vi "Actor Core.vi"(8 "error in":errorcluster, 11 "Image Averaging in":refnum<class "Image Averaging.lvclass">) -> (0 "error out":errorcluster, 3 "Actor out":refnum<class "Actor.lvclass">)   [LabVIEW 2022 SP3, in "Image Averaging.lvlib" / "Image Averaging.lvclass"]
doc: "(<B>Filename</B>: Actor Framework.lvlib:Actor.lvclass:Actor Core.vi)\n\nReceives messages to the actor, reacts to them, and initiates any error handling that may shut the actor down.\n\nDescendant classes may override this VI to append parallel tasks for the actor to complete while it handles messages. Overrides use the Call Parent Class Method node."
uses:
  Image Averaging.lvclass
  C:/Program Files/National Instruments/LabVIEW 2022/vi.lib/ActorFramework/Actor/Actor.lvclass
  <vilib>/ActorFramework/Actor/Actor.lvclass
  Image Calibration/Bontech Calibration/TypeDef/Image Averaging Image Type.ctl
  <vilib>/vision/Image Controls.llb/IMAQ Image.ctl
  Typedef/AvgStates.ctl
  Image Averaging.lvclass/Image Averaging.ctl
  BonTechDetector/Controls/Acquisition Modes.ctl
  BonTechDetector/Controls/Acquisition Commands.ctl
  <vilib>/ActorFramework/Actor/Actor.lvclass/Actor.ctl
  <vilib>/ActorFramework/Message Enqueuer/Message Enqueuer.lvclass/Message Enqueuer.ctl
  ImageHandler - Controller -- Interface/ImageHandler - Controller -- Interface Messages/Avg Done Msg/Avg Done Msg.lvclass/Avg Done Msg.ctl
  <vilib>/ActorFramework/Message Enqueuer/Enqueue.vi
  <vilib>/ActorFramework/Message Enqueuer/Init from Existing Queue.vi
  ImageHandler - Controller -- Interface/ImageHandler - Controller -- Interface Messages/Avg Done Msg/Avg Done Msg.lvclass
  C:/Program Files/National Instruments/LabVIEW 2022/vi.lib/ActorFramework/Message/Message.lvclass
  <vilib>/ActorFramework/Stop Msg/Stop Msg.lvclass
  <vilib>/ActorFramework/Message Priority Queue/Priority Enqueue.vi
  <vilib>/ActorFramework/Message Enqueuer/Message Enqueuer.lvclass
  Image Averaging.lvlib
  BonTechDetector/BonTechDetector.lvlib
  <userlib>/_MGI/Error Reporter/MGI Error Reporter Base/MGI Error Reporter Base.lvclass
panel:
  in  "Select Image Type":T1
  in  "Bright Image":bool
  in  "Dark Image":bool
  in  "No.of images":u16
  out "Progress":u16(slide) caption="Image Averaging Complete.." scale=0.0..100.0
  out "Status":string
  # "Aayvu Image Averaging Tool"
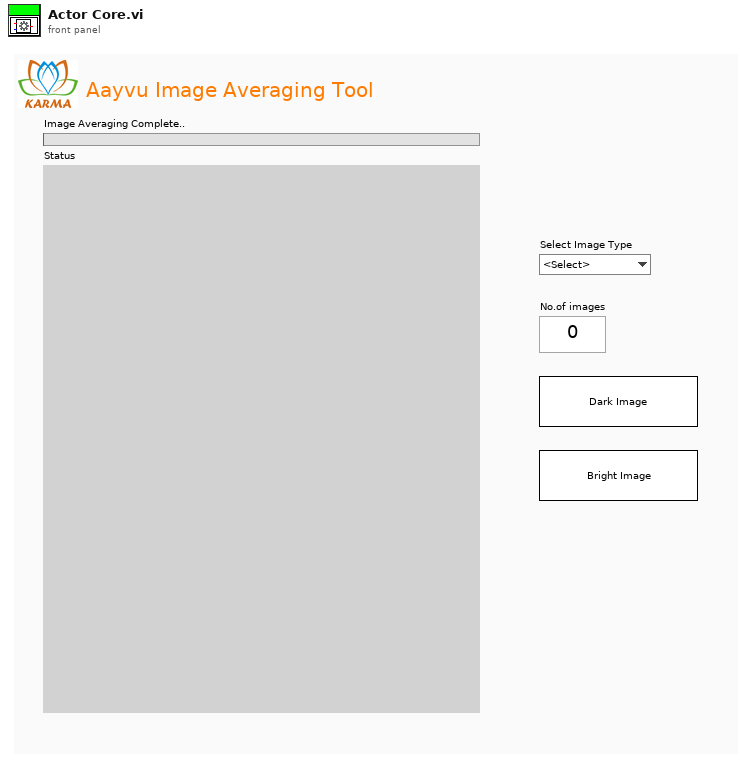
[diagram p1: front panel]
types:
  T1 = typedef "Image Averaging.lvlib/Image Averaging Image Type.ctl" = enum16{"<Select>", "TIFF", "RAW"}
  T2 = cluster{"nHostIP":string, "nSensorIP":string, "nHeight":u32, "nWidth":u32, "pImg":u16[], "refImg":u16[], "avgBuff":dbl[], "pBrightImg":u16[], "pDarkImg":u16[]}
  T3 = typedef "Image Averaging.lvlib/AvgStates.ctl" = enum16{"Poll", "Initialize", "Start Acquisition", "Get Dark Image", "Get Bright Image", "Average", "Stop Acquisition", "Save Dark Image", "Save Bright Image", "Error", "Exit"}
  T4 = typedef "IMAQ Image.ctl" = refnum<image>
  T5 = cluster{"AvgQ":refnum<queue>, "Image Data":cluster{"Img Buffer":T4, "Img Buffer1":T4, "Img U16 Buffer1":T4, "Img  u16 Buffer2":T4}, "Image Storage Path":path, "UI Data":cluster{"Img Avg Num":u16, "Progress":u16, "Status":string, "Progress 2":refnum<vi>, "Status Ref":refnum<vi>, "Iteration":u16, "Select Image Type":T1}, "AvgBuff":dbl[], "Image Averaging in":refnum<class "Image Averaging.lvclass">, "Status Event":refnum<user-event>, "U16 Buffer":T4, "Sensor Data":cluster{"nHostIP":string, "nSensorIP":string, "nHeight":i32, "nWidth":i32, "pImg":u16[], "refImg":u16[], "avgBuff":u32[], "pBrightImg":u16[], "pDarkImg":u16[], "Reference Directory":string}, "Receive Buffer":T4, "Image Pixels (U32)":u32[][]}
  T6 = cluster{"nHostIP":string, "nSensorIP":string, "nHeight":i32, "nWidth":i32, "pImg":u16[], "refImg":u16[], "avgBuff":dbl[], "pBrightImg":u16[], "pDarkImg":u16[], "Reference Directory":string}
  T7 = cluster{"Dark Img Buffer":T4, "Bright Img Buffer":T4, "U16 Dark Buffer":T4, "U16 Bright Buffer":T4}
  T8 = cluster{"Iteration":u16, "Image Out":T4, "pImg":u16[]}
  T9 = enum16{"big-endian, network order", "native, host order", "little-endian"}
  T10 = enum16{"open", "replace", "create", "open or create", "replace or create", "replace or create with confirmation"}
  T11 = typedef "Image Type" = u32
  T12 = typedef "BonTechDetector.lvlib/Acquisition Modes.ctl" = enum32{"IMAGECAP_TRIGGER_MODE", "IMAGECAP_AED_MODE", "IMAGECAP_SOFTTRIGGER_MODE", "IMAGECAP_AVG_COUNT_MODE", "IMAGECAP_AVG_AED_MODE", "IMAGECAP_CONTINUOUS_MODE", "IMAGECAP_VIEWER_MODE", "IMAGECAP_CONTINUOUS_BINNING_MODE"}
  T13 = typedef "BonTechDetector.lvlib/Acquisition Commands.ctl" = u32
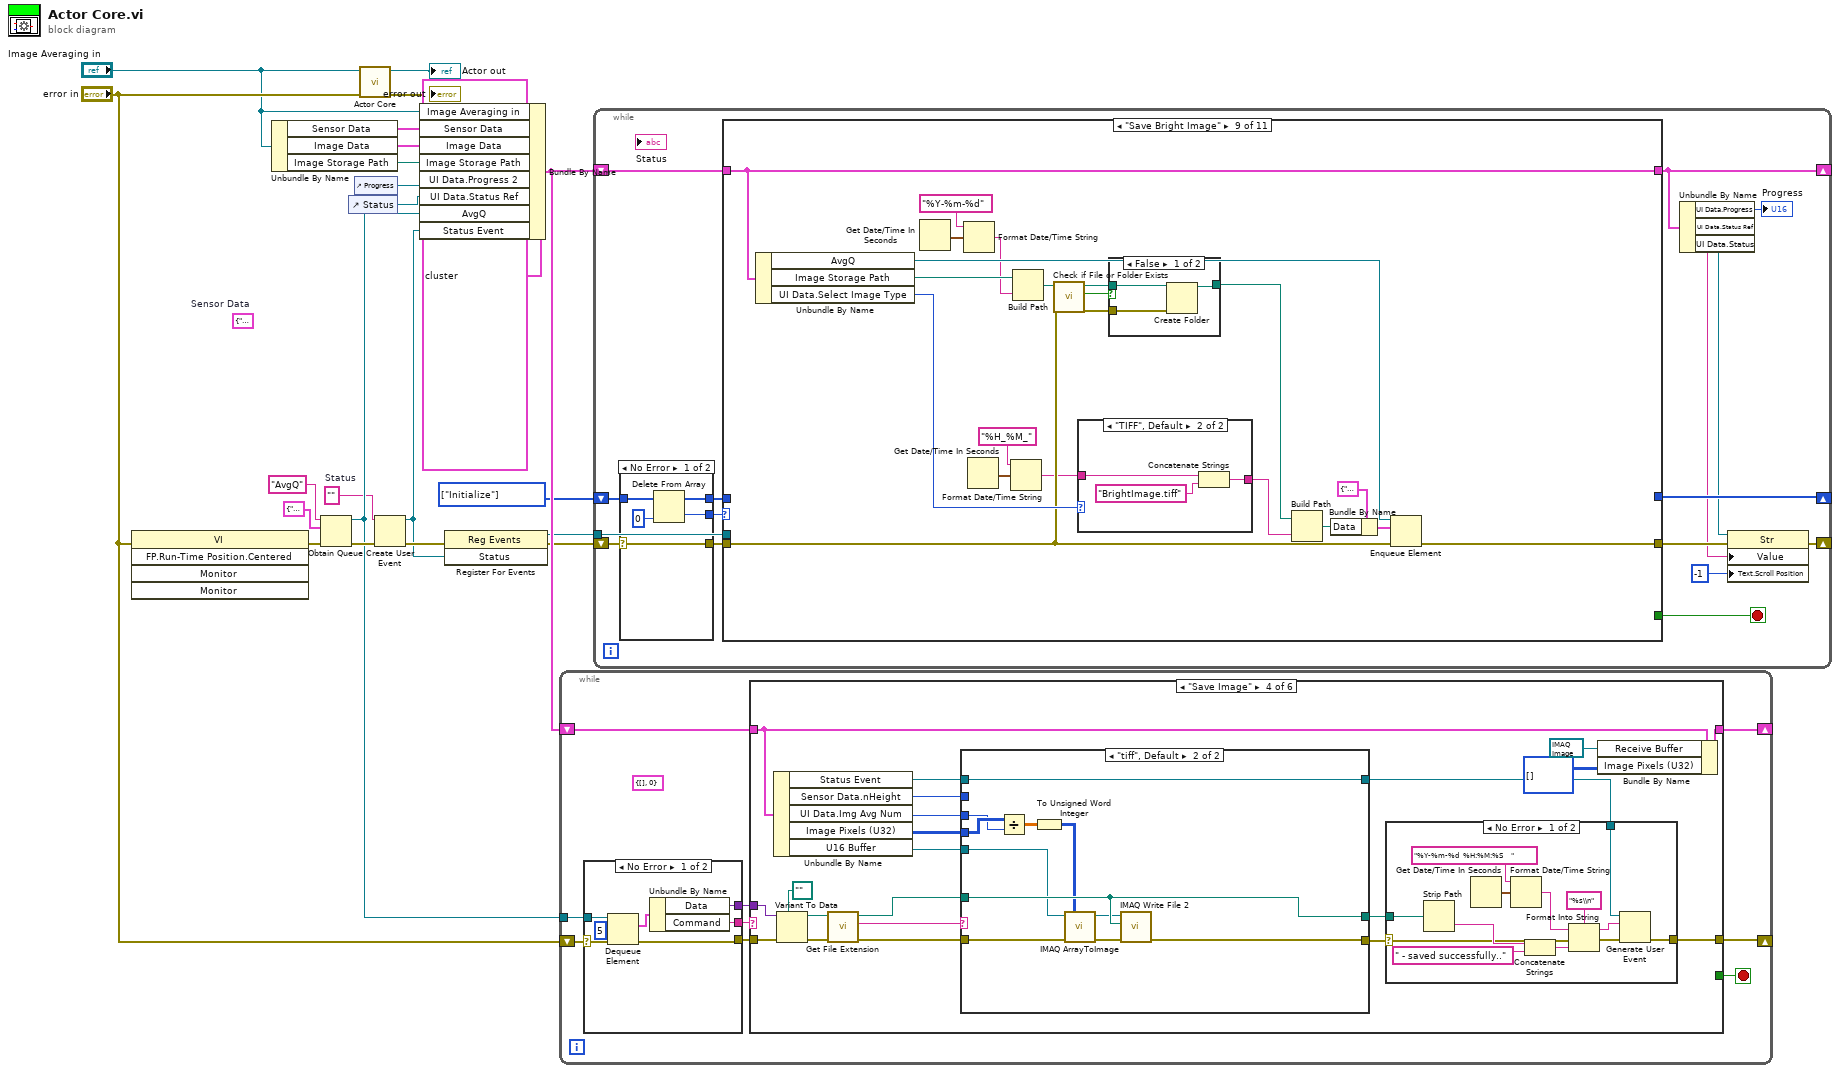
[diagram p0: block diagram]
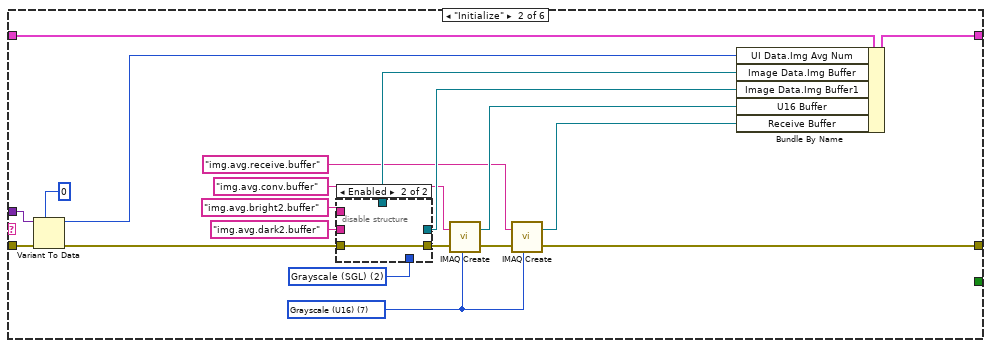
[diagram p3: hidden frame]
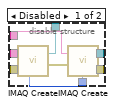
[diagram p4: hidden frame]
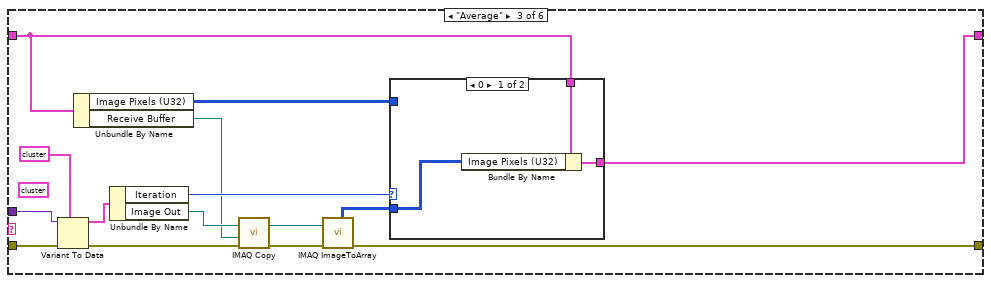
[diagram p5: hidden frame]
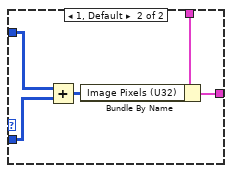
[diagram p6: hidden frame]
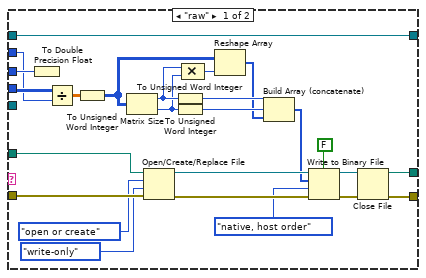
[diagram p8: hidden frame]
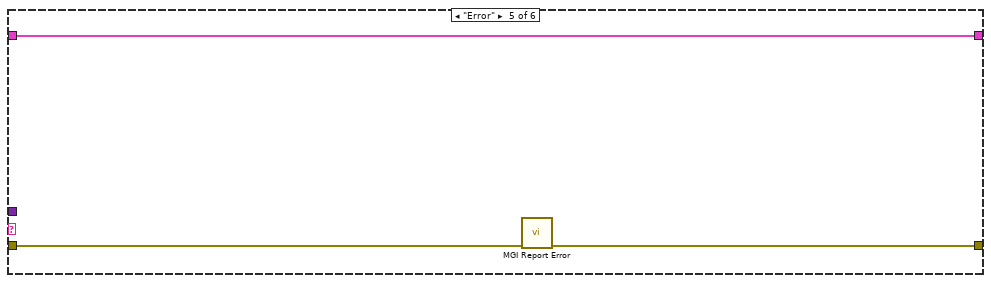
[diagram p9: hidden frame]
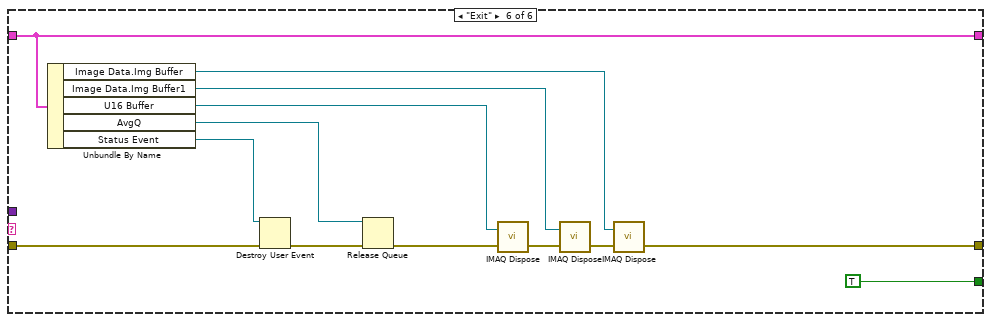
[diagram p10: hidden frame]
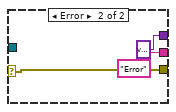
[diagram p11: hidden frame]
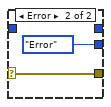
[diagram p12: hidden frame]
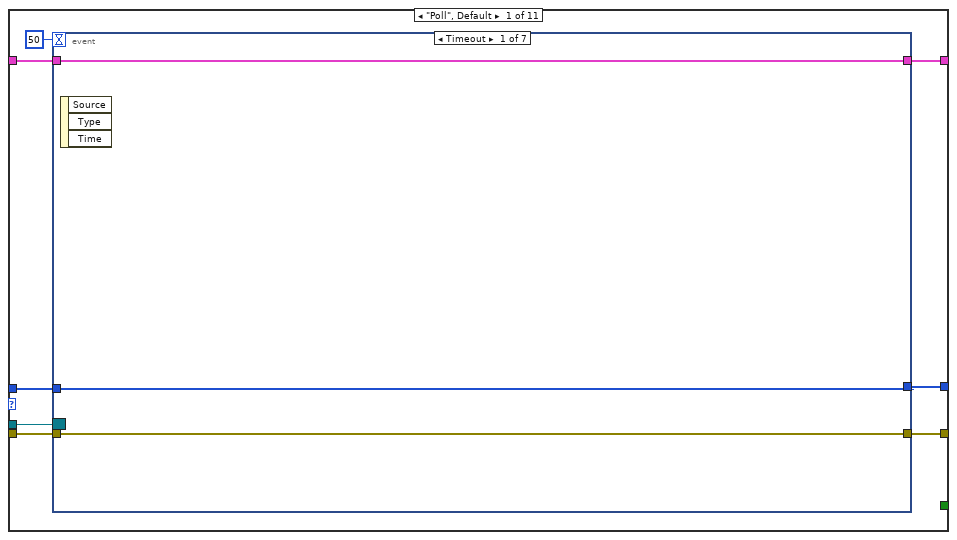
[diagram p13: hidden frame]
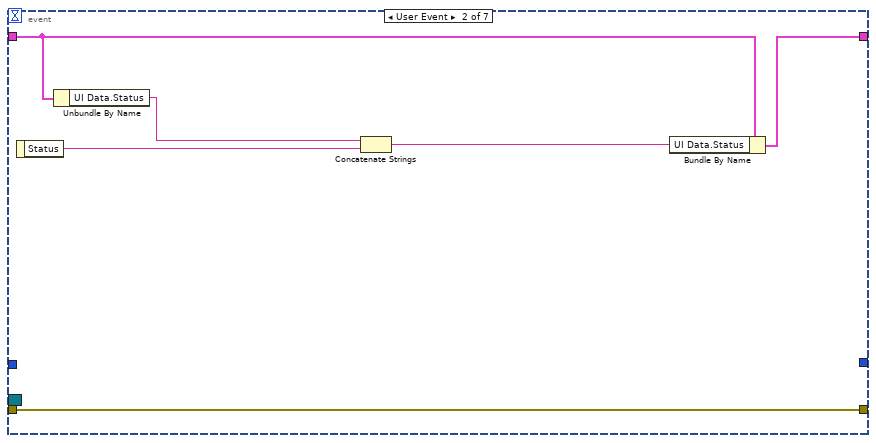
[diagram p14: hidden frame]
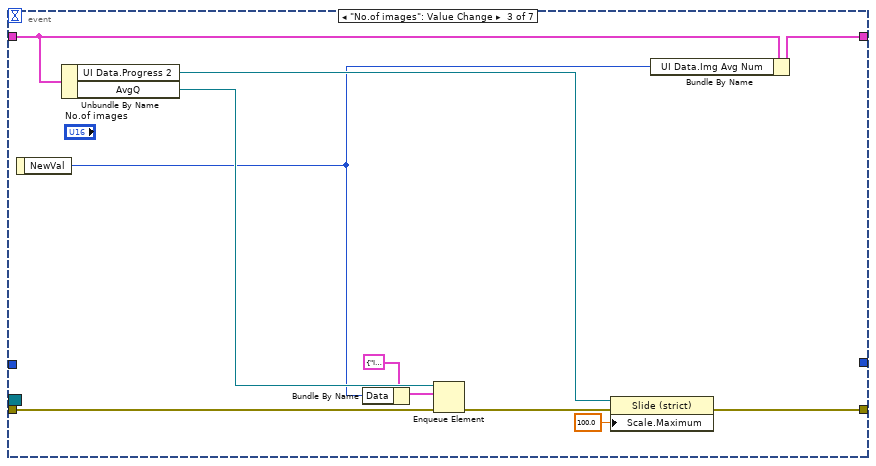
[diagram p15: hidden frame]
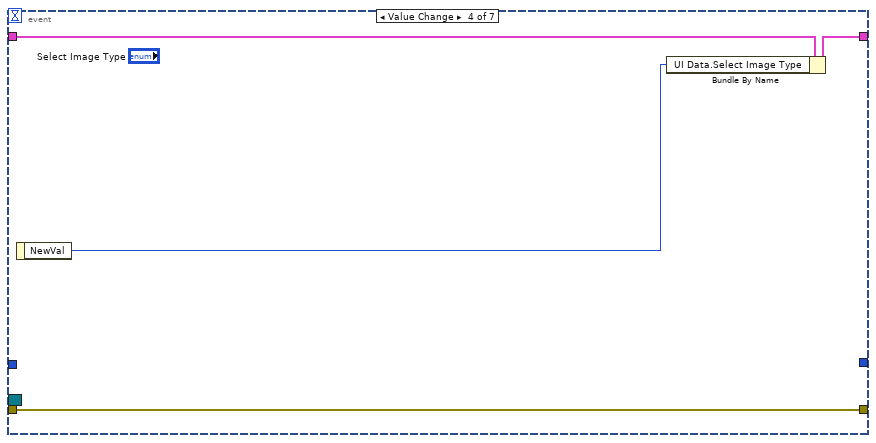
[diagram p16: hidden frame]
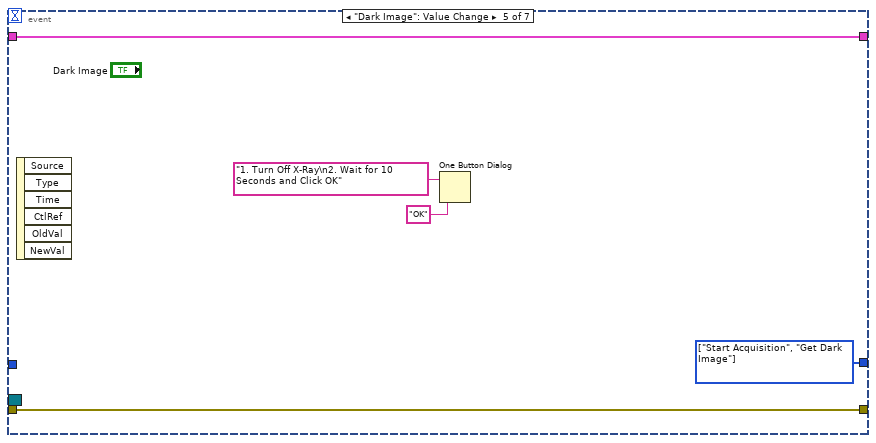
[diagram p17: hidden frame]
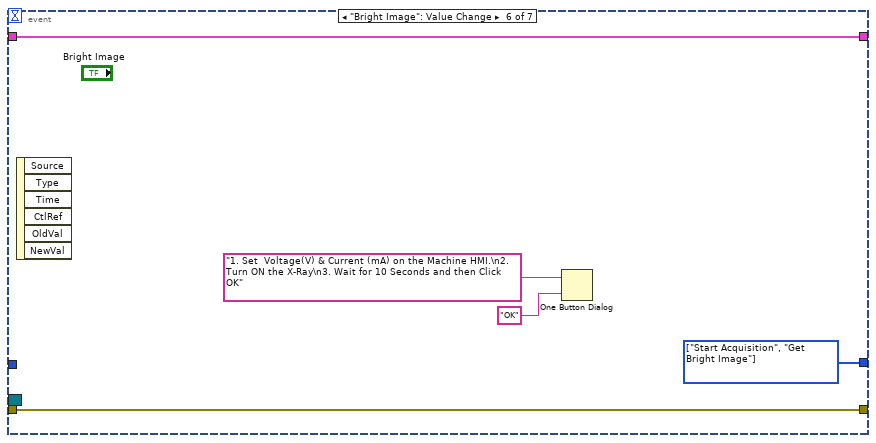
[diagram p18: hidden frame]
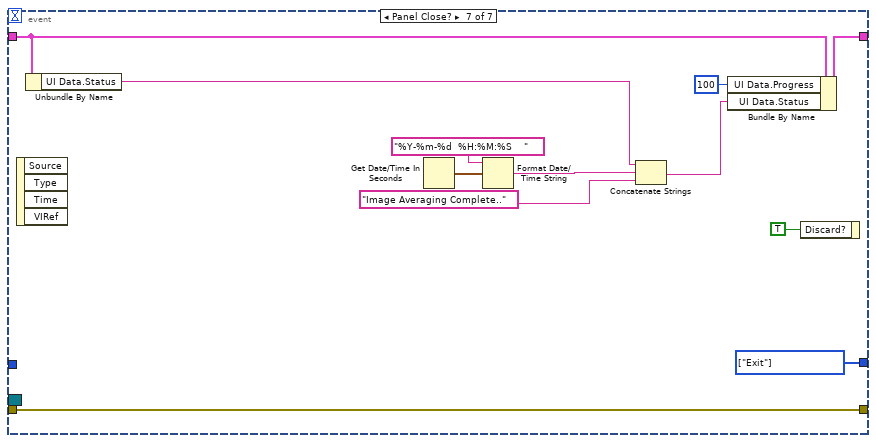
[diagram p19: hidden frame]
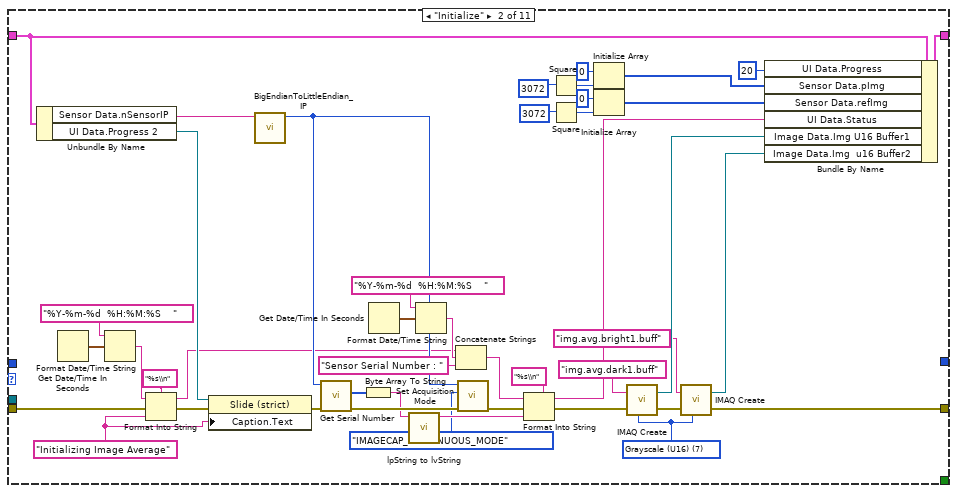
[diagram p20: hidden frame]
diagram:
  (unwired) T2 {"nHostIP"="", "nSensorIP"="", "nHeight"=0, "nWidth"=0, "pImg"=[], "refImg"=[], "avgBuff"=[], "pBrightImg"=[], "pDarkImg"=[]}  # Sensor Data
  w7 = ""  # Status
  w14 = T3[] [enum."Initialize"] items=["Poll", "Initialize", "Start Acquisition", "Get Dark Image", "Get Bright Image", "Average", "Stop Acquisition", "Save Dark Image", "Save Bright Image", "Error", "Exit"]
  n1 = invoke class="VI" method="FP.Run-Time Position.Centered"(error in="error in") -> (error out=w9:errorcluster)  [unwired: 4 in, 4 out]
  n2 = Unbundle By Name("Image Averaging in") -> ("Sensor Data"=w1:T6, "Image Data"=w2:T7, "Image Storage Path"=w3:path)
  n3 = Obtain Queue(name (unnamed)="AvgQ", element data type=cluster{"Command":string, "Data":variant} {"Command"="", "Data"=variant}, error in (no error)=w9) -> (queue out=w13:refnum<queue>, error out=w19:errorcluster)  [unwired: 2 in, 1 out]
  n4 = control-ref of="Status"() -> (w11:refnum<vi>)
  n5 = control-ref of="Progress"() -> (w12:refnum<vi>)
  n6 = call-parent "Actor Core.vi"("error in"="error in", "Actor in"="Image Averaging in") -> ("error out"=→"error out":errorcluster, "Actor out"=→"Actor out":refnum<class "Actor.lvclass">)  [unwired: 8 in]
  n7 = Create User Event(user event datatype=w7, error in=w19) -> (user event=w4:refnum<user-event>, error out=w8:errorcluster)
  n8 = Bundle By Name(cluster=T5 {"AvgQ"=refnum, "Image Data"={"Img Buffer"=refnum, "Img Buffer1"=refnum, "Img U16 Buffer1"=refnum, "Img  u16 Buffer2"=refnum}, "Image Storage Path"=path "", "UI Data"={"Img Avg Num"=0, "Progress"=0, "Status"="", "Progress 2"=refnum, "Status Ref"=refnum, "Iteration"=0, "Select Image Type"=enum."<Select>"}, "AvgBuff"=[], "Image Averaging in"=refnum, "Status Event"=refnum, "U16 Buffer"=refnum, "Sensor Data"={"nHostIP"="", "nSensorIP"="", "nHeight"=0, "nWidth"=0, "pImg"=[], "refImg"=[], "avgBuff"=[], "pBrightImg"=[], "pDarkImg"=[], "Reference Directory"=""}, "Receive Buffer"=refnum, "Image Pixels (U32)"=[]}, "Image Averaging in"="Image Averaging in", "Sensor Data"=w1, "Image Data"=w2, "Image Storage Path"=w3, "UI Data.Progress 2"=w12, "UI Data.Status Ref"=w11, "AvgQ"=w13, "Status Event"=w4) -> (w15:T5)
  n9 = register-events(error in=w8, w4) -> (reference out=w5:refnum<event-registration>, error out=w6:errorcluster)  [unwired: 1 in]
  n10 = while {
    shift-right: [w23] -> _
    shift-left: w15 -> [w29]
    shift-right: [w25] -> _
    shift-left: "error in" -> [w31]
    tunnel: w13 -> [w30]
    stop <- w24 stop-if-true
    (unwired) cluster{"pImg":u16[], "Iteration":u16} {"pImg"=[], "Iteration"=0}
    n11 = case shown="No Error" w31 {
      selector: w31 -> [w179 w181]
      tunnel: w30 -> [w178 _]
      tunnel: [w176 "Error" ("Command")] -> w28
      tunnel: [w175 w181] -> w27
      tunnel: [w174 variant ("Data")] -> w26
      frame No Error {
        n12 = Dequeue Element(queue=w178, timeout in ms (-1)=5, error in (no error)=w179) -> (element=w177:cluster{"Command":string, "Data":variant}, error out=w175:errorcluster)  [unwired: 2 out]
        n13 = Unbundle By Name(w177) -> ("Data"=w174:variant, "Command"=w176:string)
      }
      frame Error {
      }
    }
    n14 = case shown="\"Save Image\"" w28 {
      tunnel: w29 -> [w32 w53 w73 w104 w158 w169]
      tunnel: [w32 w48 w72 w88 w158 w169] -> w23
      tunnel: w27 -> [w33 w52 w77 w106 w159 w172]
      tunnel: w26 -> [_ w50 w76 w105 _ _]
      tunnel: [w33 w37 w63 w96 w157 w164] -> w25
      tunnel: [_ _ _ _ _ TRUE] -> w24
      frame "Poll", Default {
      }
      frame "Initialize" {
        w35 = T11 7 items=["Grayscale (U8)", "Grayscale (I16)", "Grayscale (SGL)", "Complex (CSG)", "RGB (U32)", "HSL (U32)", "RGB (U64)", "Grayscale (U16)"] ("Image Type")
        w43 = T11 2 items=["Grayscale (U8)", "Grayscale (I16)", "Grayscale (SGL)", "Complex (CSG)", "RGB (U32)", "HSL (U32)", "RGB (U64)", "Grayscale (U16)"] ("Image Type")
        n15 = Variant To Data(error in=w52, type=u16 0 ("NewVal"), Variant=w50) -> (data=w47:u16, error out=w51:errorcluster)
        n16 = disable-structure shown="Enabled" {
          disable-tunnel: w51 -> [w61 w62]
          disable-tunnel: [w59 w62] -> w49
          disable-tunnel: [w58 _] -> w45
          disable-tunnel: [w57 _] -> w44
          disable-tunnel: w43 -> [w56 _]
          disable-tunnel: "img.avg.dark2.buffer" ("Image Name") -> [w55 _]
          disable-tunnel: "img.avg.bright2.buffer" ("Image Name") -> [w54 _]
          frame Disabled {
            n17 = call "IMAQ Create"("Image Name"=w55, "Image Type"=w56, "error in (no error)"=w61) -> ("New Image"=w58:T4, "error out"=w60:errorcluster)  [unwired: 2 in]
            n18 = call "IMAQ Create"("Image Name"=w54, "Image Type"=w56, "error in (no error)"=w60) -> ("New Image"=w57:T4, "error out"=w59:errorcluster)  [unwired: 2 in]
          }
          frame Enabled {
          }
        }
        n19 = call "IMAQ Create"("Image Name"="img.avg.conv.buffer", "Image Type"=w35, "error in (no error)"=w49) -> ("New Image"=w38:T4, "error out"=w40:errorcluster)  [unwired: 2 in]
        n20 = call "IMAQ Create"("Image Name"="img.avg.receive.buffer", "Image Type"=w35, "error in (no error)"=w40) -> ("New Image"=w34:T4, "error out"=w37:errorcluster)  [unwired: 2 in]
        n21 = Bundle By Name(cluster=w53, "UI Data.Img Avg Num"=w47, "Image Data.Img Buffer"=w45, "Image Data.Img Buffer1"=w44, "U16 Buffer"=w38, "Receive Buffer"=w34) -> (w48:T5)
      }
      frame "Average" {
        (unwired) cluster{"Iteration":u16, "Image Out":T4} {"Iteration"=0, "Image Out"=refnum}
        n22 = Variant To Data(error in=w77, type=T8 {"Iteration"=0, "Image Out"=refnum, "pImg"=[]}, Variant=w76) -> (data=w75:T8, error out=w71:errorcluster)
        n23 = Unbundle By Name(w73) -> ("Image Pixels (U32)"=w74:u32[][], "Receive Buffer"=w67:T4)
        n24 = Unbundle By Name(w75) -> ("Iteration"=w68:u16, "Image Out"=w69:T4)
        n25 = call "IMAQ Copy"("error in (no error)"=w71, "Image Dst"=w67, "Image Src"=w69) -> ("error out"=w70:errorcluster, "Image Dst Out"=w65:T4)  [unwired: 3 in]
        n26 = call "IMAQ ImageToArray"("error in (no error)"=w70, "Image"=w65) -> ("Image Pixels (U16)"=w64:u16[][], "error out"=w63:errorcluster)  [unwired: 2 in, 3 out]
        n27 = case shown="0" w68 {
          tunnel: w74 -> [_ w83]
          tunnel: w73 -> [w80 w85]
          tunnel: [w79 w84] -> w72
          tunnel: w64 -> [w78 w82]
          frame 0 {
            n28 = Bundle By Name(cluster=w80, "Image Pixels (U32)"=w78) -> (w79:T5)
          }
          frame 1, Default {
            n29 = Add(x=w83, y=w82) -> (x+y=w81:u32[][])
            n30 = Bundle By Name(cluster=w85, "Image Pixels (U32)"=w81) -> (w84:T5)
          }
        }
      }
      frame "Save Image" {
        n31 = Unbundle By Name(w104) -> ("Status Event"=w95:refnum<user-event>, "Sensor Data.nHeight"=w89:i32, "UI Data.Img Avg Num"=w91:u16, "Image Pixels (U32)"=w92:u32[][], "U16 Buffer"=w90:T4)
        n32 = Variant To Data(error in=w106, type=path "" ("appended path"), Variant=w105) -> (data=w100:path, error out=w103:errorcluster)
        n33 = call <vilib>:"Get File Extension.vi"("error in (no error)"=w103, "file"=w100) -> ("error out"=w101:errorcluster, "lowercase file extension"=w98:string, "dup file"=w99:path)  [unwired: 5 in, 2 out]
        n34 = case shown="\"tiff\", Default" w98 {
          tunnel: [w136 w156] -> w93
          tunnel: w101 -> [w145 w155]
          tunnel: w99 -> [w144 w154]
          tunnel: [w135 w154] -> w97
          tunnel: w95 -> [w134 w153]
          tunnel: [w134 w153] -> w94
          tunnel: w92 -> [w124 w151]
          tunnel: w91 -> [w133 w150]
          tunnel: w90 -> [_ w147]
          tunnel: w89 -> [w123 _]
          frame "raw" {
            n35 = To Double Precision Float(number=w133) -> ()  [unwired: 1 out]
            n36 = Divide(x=w124, y=w123) -> (x/y=w122:dbl[][])
            n37 = To Unsigned Word Integer(number=w122) -> (unsigned 16bit integer=w121:u16[][])
            n38 = Matrix Size(0:w121) -> (1:w128:i32, 2:w127:i32)
            n39 = Open/Create/Replace File(file path (use dialog)=w144, error in=w145, operation (0:open)=T10."open or create", access (0:read/write)=enum16{"read/write", "read-only", "write-only"}."write-only") -> (refnum out=w140:refnum<file>, error out=w141:errorcluster)  [unwired: 2 in, 1 out]
            n40 = To Unsigned Word Integer(number=w128) -> (unsigned 16bit integer=w131:u16)
            n41 = To Unsigned Word Integer(number=w127) -> (unsigned 16bit integer=w130:u16)
            n42 = Compound Arithmetic op=MULTIPLY(w128, w127) -> (w132:i32)
            n43 = Reshape Array(w121, w132) -> (w125:u16[])
            n44 = Build Array (concatenate)(w131, w130, w125) -> (w129:u16[])
            n45 = Write to Binary File(file (use dialog)=w140, data=w129, error in=w141, 5:FALSE ("prepend array or string size? (T)"), 9:T9."native, host order" ("byte order (0:big-endian, network order)")) -> (refnum out=w138:refnum<file>, error out=w137:errorcluster)  [unwired: 1 in, 1 out]
            n46 = Close File(refnum=w138, error in=w137) -> (path=w135:path, error out=w136:errorcluster)
          }
          frame "tiff", Default {
            n47 = Divide(x=w151, y=w150) -> (x/y=w149:dbl[][])
            n48 = To Unsigned Word Integer(number=w149) -> (unsigned 16bit integer=w148:u16[][])
            n49 = call "IMAQ ArrayToImage"("Image Pixels (U16)"=w148, "error in (no error)"=w155, "Image"=w147) -> ("error out"=w152:errorcluster, "Image Out"=w146:T4)  [unwired: 7 in]
            n50 = call-poly "IMAQ Write File 2"("error in (no error)"=w152, "File Path"=w154, "Image"=w146) -> ("error out"=w156:errorcluster)  [unwired: 7 in, 1 out]
          }
        }
        n51 = case shown="No Error" w93 {
          selector: w93 -> [w107 w120]
          tunnel: w97 -> [w112 _]
          tunnel: [w110 w120] -> w96
          tunnel: w94 -> [w108 _]
          frame No Error {
            n52 = Strip Path(path=w112) -> (name=w111:string)  [unwired: 1 out]
            n53 = Get Date/Time In Seconds() -> (seconds since 1Jan1904=w119:timestamp)
            n54 = Format Date/Time String(time format string (%c)="%Y-%m-%d  %H:%M:%S    ", seconds (now)=w119) -> (date/time string=w117:string)  [unwired: 1 in]
            n55 = Concatenate Strings(w111, " - saved successfully.." ("string")) -> (w115:string)
            n56 = Format Into String(format string="%s\\n", initial string=w117, error in=w107, w115) -> (resulting string=w109:string, error out=w113:errorcluster)
            n57 = Generate User Event(user event=w108, event data cluster=w109, error in=w113) -> (error out=w110:errorcluster)  [unwired: 1 in, 1 out]
          }
          frame Error {
          }
        }
        n58 = Bundle By Name(cluster=w104, "Receive Buffer"=T4 refnum, "Image Pixels (U32)"=u32[][] []) -> (w88:T5)
      }
      frame "Error" {
        n59 = call <userlib>:"MGI Report Error.vi"("error in"=w159) -> ("no error"=w157:errorcluster)  [unwired: 10 in]
      }
      frame "Exit" {
        n60 = Unbundle By Name(w169) -> ("Image Data.Img Buffer"=w160:T4, "Image Data.Img Buffer1"=w161:T4, "U16 Buffer"=w162:T4, "AvgQ"=w168:refnum<queue>, "Status Event"=w166:refnum<user-event>)
        n61 = Destroy User Event(user event=w166, error in=w172) -> (error out=w167:errorcluster)
        n62 = Release Queue(queue=w168, error in (no error)=w167) -> (error out=w170:errorcluster)  [unwired: 1 in, 2 out]
        n63 = call "IMAQ Dispose"("Image"=w162, "error in (no error)"=w170) -> ("error out"=w163:errorcluster)  [unwired: 4 in]
        n64 = call "IMAQ Dispose"("Image"=w161, "error in (no error)"=w163) -> ("error out"=w165:errorcluster)  [unwired: 4 in]
        n65 = call "IMAQ Dispose"("Image"=w160, "error in (no error)"=w165) -> ("error out"=w164:errorcluster)  [unwired: 4 in]
      }
    }
  }
  n66 = while {
    shift-right: [w189] -> _
    shift-left: w15 -> [w198]
    shift-right: [w187] -> _
    shift-left: w6 -> [w197]
    shift-right: [w191] -> _
    shift-left: w14 -> [w196]
    tunnel: w5 -> [w183]
    stop <- w190 stop-if-true
    n67 = case shown="No Error" w197 {
      selector: w197 -> [w199 w205]
      tunnel: w196 -> [w203 _]
      tunnel: [w201 AvgStates."Error" ("Enum")] -> w195
      tunnel: [w200 _] -> w194
      tunnel: [w199 w205] -> w193
      frame No Error {
        n68 = Delete From Array(array=w203, index=0) -> (deleted portion=w201:T3, array with subset deleted=w200:T3[])  [unwired: 1 in]
      }
      frame Error {
      }
    }
    n69 = case shown="\"Save Bright Image\"" w195 {
      tunnel: w198 -> [w213 w288 w320 w333 w412 w481 w485 w507 w538 w555 w581]
      tunnel: [w212 w303 w312 w332 w411 w481 w485 w507 w538 w552 w569] -> w189
      tunnel: w194 -> [w209 _ w306 _ _ _ w482 _ _ _ _]
      tunnel: w193 -> [w210 w290 w321 w340 w419 w480 w487 w500 w531 w554 w582]
      tunnel: [w207 w267 w313 w339 w418 w480 w486 w508 w539 w553 w566] -> w192
      tunnel: [w208 _ w306 w325 w404 _ w482 _ _ _ _] -> w191
      tunnel: [_ _ _ _ _ _ _ _ _ _ TRUE] -> w190
      tunnel: w183 -> [w206 _ _ _ _ _ _ _ _ _ w562]
      frame "Poll", Default {
        n70 = event shown="[0] Timeout" {
          selector: w206 -> [_ _ _ _ _ _ _]
          dyn-events: _ -> [_ _ _ _ _ _ _]
          timeout: 50 -> [_ _ _ _ _ _ _]
          tunnel: w213 -> [w216 w218 w230 w237 w242 w247 w252]
          tunnel: [w216 w221 w232 w235 w242 w247 w250] -> w212
          tunnel: w210 -> [w214 w222 w233 w236 w241 w246 w259]
          tunnel: [w215 _ _ _ w240 w245 w257] -> w208
          tunnel: w209 -> [w215 _ _ _ _ _ _]
          tunnel: [w214 w222 w226 w236 w241 w246 w259] -> w207
          event Timeout {
            n71 = event-data() -> ()  [unwired: 1 in, 3 out]
          }
          event User Event {
            n72 = event-data() -> ("Status"=w220:string)  [unwired: 1 in]
            n73 = Unbundle By Name(w218) -> ("UI Data.Status"=w217:string)
            n74 = Concatenate Strings(w217, w220) -> (w219:string)
            n75 = Bundle By Name(cluster=w218, "UI Data.Status"=w219) -> (w221:T5)
          }
          event "No.of images": Value Change {
            n76 = event-data() -> ("NewVal"=w224:u16)  [unwired: 1 in]
            n77 = Unbundle By Name(w230) -> ("UI Data.Progress 2"=w225:refnum<vi>, "AvgQ"=w229:refnum<queue>)
            n78 = Bundle By Name(cluster=cluster{"Command":string, "Data":variant} {"Command"="Initialize", "Data"=variant} ("element"), "Data"=w224) -> (w227:cluster{"Command":string, "Data":variant})
            n79 = Enqueue Element(queue=w229, element=w227, error in (no error)=w233) -> (error out=w231:errorcluster)  [unwired: 1 in, 2 out]
            n80 = property class="Slide (strict)"(reference=w225, error in=w231, "Scale.Maximum"=100.0 ("Scale.Range:Maximum")) -> (error out=w226:errorcluster)  [unwired: 1 out]
            n81 = Bundle By Name(cluster=w230, "UI Data.Img Avg Num"=w224) -> (w232:T5)
          }
          event Value Change {
            n82 = event-data() -> ("NewVal"=w234:T1)  [unwired: 1 in]
            n83 = Bundle By Name(cluster=w237, "UI Data.Select Image Type"=w234) -> (w235:T5)
          }
          event "Dark Image": Value Change {
            w240 = T3[] [enum."Start Acquisition", enum."Get Dark Image"] items=["Poll", "Initialize", "Start Acquisition", "Get Dark Image", "Get Bright Image", "Average", "Stop Acquisition", "Save Dark Image", "Save Bright Image", "Error", "Exit"]
            n84 = event-data() -> ()  [unwired: 1 in, 6 out]
            n85 = One Button Dialog(message="1. Turn Off X-Ray\n2. Wait for 10 Seconds and Click OK", button name ("OK")="OK") -> ()  [unwired: 1 out]
          }
          event "Bright Image": Value Change {
            w245 = T3[] [enum."Start Acquisition", enum."Get Bright Image"] items=["Poll", "Initialize", "Start Acquisition", "Get Dark Image", "Get Bright Image", "Average", "Stop Acquisition", "Save Dark Image", "Save Bright Image", "Error", "Exit"]
            n86 = event-data() -> ()  [unwired: 1 in, 6 out]
            n87 = One Button Dialog(message="1. Set  Voltage(V) & Current (mA) on the Machine HMI.\n2. Turn ON the X-Ray\n3. Wait for 10 Seconds and then Click OK", button name ("OK")="OK") -> ()  [unwired: 1 out]
          }
          event Panel Close? {
            w257 = T3[] [enum."Exit"] items=["Poll", "Initialize", "Start Acquisition", "Get Dark Image", "Get Bright Image", "Average", "Stop Acquisition", "Save Dark Image", "Save Bright Image", "Error", "Exit"]
            n88 = event-data() -> ()  [unwired: 1 in, 4 out]
            n89 = Unbundle By Name(w252) -> ("UI Data.Status"=w251:string)
            n90 = Get Date/Time In Seconds() -> (seconds since 1Jan1904=w256:timestamp)
            n91 = Format Date/Time String(time format string (%c)="%Y-%m-%d  %H:%M:%S    ", seconds (now)=w256) -> (date/time string=w254:string)  [unwired: 1 in]
            n92 = Concatenate Strings(w251, w254, "Image Averaging Complete.." ("string")) -> (w249:string)
            n93 = Bundle By Name(cluster=w252, "UI Data.Progress"=u16 100, "UI Data.Status"=w249) -> (w250:T5)
            n94 = event-data("Discard?"=TRUE) -> ()  [unwired: 1 in, 1 out]
          }
        }
      }
      frame "Initialize" {
        w262 = T11 7 items=["Grayscale (U8)", "Grayscale (I16)", "Grayscale (SGL)", "Complex (CSG)", "RGB (U32)", "HSL (U32)", "RGB (U64)", "Grayscale (U16)"] ("Image Type")
        w276 = "Initializing Image Average" ("input 1")
        n95 = Unbundle By Name(w288) -> ("Sensor Data.nSensorIP"=w287:string, "UI Data.Progress 2"=w277:refnum<vi>)
        n96 = Get Date/Time In Seconds() -> (seconds since 1Jan1904=w294:timestamp)
        n97 = Format Date/Time String(time format string (%c)="%Y-%m-%d  %H:%M:%S    ", seconds (now)=w294) -> (date/time string=w292:string)  [unwired: 1 in]
        n98 = Format Into String(format string="%s\\n", initial string=w292, error in=w290, w276) -> (resulting string=w274:string, error out=w289:errorcluster)
        n99 = property class="Slide (strict)"(reference=w277, error in=w289, "Caption.Text"=w276) -> (error out=w278:errorcluster)  [unwired: 1 out]
        n100 = call "BigEndianToLittleEndian_IP.vi"("IP String"=w287) -> ("IP Network Order"=w280:u32)  [unwired: 10 in]
        n101 = call "Get Serial Number.vi"("error in (no error)"=w278, "nSensorIP"=w280) -> ("error out"=w272:errorcluster, "lpszSerialNum out"=w271:u8[])  [unwired: 7 in, 1 out]
        n102 = Byte Array To String(unsigned byte array=w271) -> (string=w270:string)
        n103 = Get Date/Time In Seconds() -> (seconds since 1Jan1904=w285:timestamp)
        n104 = call "lpString to lvString.vi"("LPTSTR String"=w270) -> ("LVString"=w282:string)  [unwired: 10 in]
        n105 = Format Date/Time String(time format string (%c)="%Y-%m-%d  %H:%M:%S    ", seconds (now)=w285) -> (date/time string=w275:string)  [unwired: 1 in]
        n106 = Concatenate Strings(w274, w275, "Sensor Serial Number : " ("string")) -> (w261:string)
        n107 = call "Set Acquisition Mode.vi"("error in (no error)"=w272, "nMode"=Acquisition_Modes."IMAGECAP_CONTINUOUS_MODE", "nSensorIP"=w280) -> ("error out"=w281:errorcluster)  [unwired: 7 in, 1 out]
        n108 = Format Into String(format string="%s\\n", initial string=w261, error in=w281, w282) -> (resulting string=w279:string, error out=w284:errorcluster)
        n109 = Square(x=3072 ("dimension size")) -> (x^2=w300:i32)
        n110 = Square(x=3072 ("dimension size")) -> (x^2=w297:i32)
        n111 = Initialize Array(u16 0 ("element"), w300) -> (w296:u16[])
        n112 = Initialize Array(u16 0 ("element"), w297) -> (w295:u16[])
        n113 = call "IMAQ Create"("Image Name"="img.avg.dark1.buff", "Image Type"=w262, "error in (no error)"=w284) -> ("New Image"=w266:T4, "error out"=w268:errorcluster)  [unwired: 2 in]
        n114 = call "IMAQ Create"("Image Name"="img.avg.bright1.buff", "Image Type"=w262, "error in (no error)"=w268) -> ("New Image"=w265:T4, "error out"=w267:errorcluster)  [unwired: 2 in]
        n115 = Bundle By Name(cluster=w288, "UI Data.Progress"=u16 20, "Sensor Data.pImg"=w296, "Sensor Data.refImg"=w295, "UI Data.Status"=w279, "Image Data.Img U16 Buffer1"=w266, "Image Data.Img  u16 Buffer2"=w265) -> (w303:T5)
      }
      frame "Start Acquisition" {
        w304 = T13 1 items=["ACQ_INIT"=0, "DARK_MODE"=1, "BRIGHT_MODE"=2, "SOFTTRIGGER_MODE"=258, "SOFTTRIGGER_INSTANT_MODE"=259] ("nCmd")
        n116 = Unbundle By Name(w320) -> ("UI Data.Status"=w311:string, "Sensor Data.nSensorIP"=w319:string)
        n117 = call "BigEndianToLittleEndian_IP.vi"("IP String"=w319) -> ("IP Network Order"=w318:u32)  [unwired: 10 in]
        n118 = call "Send Capture Command.vi"("error in (no error)"=w321, "nCmd"=w304, "nSensorIP"=w318) -> ("error out"=w314:errorcluster)  [unwired: 7 in, 1 out]
        n119 = Get Date/Time In Seconds() -> (seconds since 1Jan1904=w308:timestamp)
        n120 = Format Date/Time String(time format string (%c)="%Y-%m-%d  %H:%M:%S    ", seconds (now)=w308) -> (date/time string=w317:string)  [unwired: 1 in]
        n121 = Format Into String(format string="%s\\n", initial string=w317, error in=w314, "Sending Capture Command" ("input 1")) -> (resulting string=w310:string, error out=w313:errorcluster)
        n122 = Concatenate Strings(w311, w310) -> (w309:string)
        n123 = Bundle By Name(cluster=w320, "UI Data.Iteration"=u16 0 ("UI Data.Progress"), "UI Data.Status"=w309) -> (w312:T5)
      }
      frame "Get Dark Image" {
        n124 = Unbundle By Name(w333) -> ("UI Data.Progress"=w331:u16, "UI Data.Status"=w329:string, "UI Data.Progress 2"=w326:refnum<vi>, "AvgQ"=w328:refnum<queue>, "UI Data.Iteration"=w330:u16, "UI Data.Img Avg Num"=w327:u16, "Image Data.Img U16 Buffer1"=w324:T4, "Sensor Data.nSensorIP"=w337:string, "Sensor Data.refImg"=w336:u16[], "Sensor Data.pImg"=w335:u16[], "Sensor Data.nHeight"=w334:i32, "Sensor Data.nWidth"=w323:i32, "Sensor Data.Reference Directory"=w322:string)
        n125 = Greater Or Equal?(x=w330, y=w327) -> (x >= y?=w338:bool)
        n126 = case shown="False" w338 {
          tunnel: w340 -> [w387 w400]
          tunnel: [w369 w400] -> w339
          tunnel: w337 -> [w384 _]
          tunnel: w336 -> [w385 _]
          tunnel: w335 -> [w386 _]
          tunnel: w334 -> [w346 _]
          tunnel: w330 -> [w371 w390]
          tunnel: w333 -> [w377 w399]
          tunnel: [w376 w398] -> w332
          tunnel: w331 -> [w357 _]
          tunnel: w329 -> [w361 w394]
          tunnel: w328 -> [w382 _]
          tunnel: w327 -> [w370 _]
          tunnel: w326 -> [w368 _]
          tunnel: [w367 w389] -> w325
          tunnel: w324 -> [w351 _]
          tunnel: w323 -> [w347 _]
          tunnel: w322 -> [w345 _]
          frame False {
            w356 = T13 1 items=["ACQ_INIT"=0, "DARK_MODE"=1, "BRIGHT_MODE"=2, "SOFTTRIGGER_MODE"=258, "SOFTTRIGGER_INSTANT_MODE"=259] ("nMode")
            w367 = T3[] [enum."Poll", enum."Get Dark Image"] items=["Poll", "Initialize", "Start Acquisition", "Get Dark Image", "Get Bright Image", "Average", "Stop Acquisition", "Save Dark Image", "Save Bright Image", "Error", "Exit"]
            n127 = call "BigEndianToLittleEndian_IP.vi"("IP String"=w384) -> ("IP Network Order"=w383:u32)  [unwired: 10 in]
            n128 = call "lvString to lpString.vi"("LVString"=w345) -> ("LPTSTR String"=w344:string)  [unwired: 10 in]
            n129 = Compound Arithmetic op=MULTIPLY(w346, w347, 2 ("value")) -> (w349:i32)
            n130 = String To Byte Array(string=w344) -> (unsigned byte array=w343:u8[])
            n131 = To Unsigned Long Integer(number=w349) -> (unsigned 32bit integer=w350:u32)
            n132 = call "Start Continuous Acquisition.vi"("nSensorIP"=w383, "nMode"=w356, "refImg"=w385, "pImg"=w386, "nBuffLength"=w350, "error in (no error)"=w387, "lpszRefPath"=w343) -> ("pImg out"=w342:u16[], "error out"=w353:errorcluster)  [unwired: 5 in, 2 out]
            n133 = Reshape Array(w342, w347, w346) -> (w354:u16[][])
            n134 = call "IMAQ ArrayToImage"("Image Pixels (U16)"=w354, "error in (no error)"=w353, "Image"=w351) -> ("error out"=w352:errorcluster, "Image Out"=w341:T4)  [unwired: 7 in]
            n135 = Decrement(x=w370) -> (x-1=w358:u16)
            n136 = Increment(x=w371) -> (x+1=w359:u16)
            n137 = Bundle By Name(cluster=T8 {"Iteration"=0, "Image Out"=refnum, "pImg"=[]}, "Iteration"=w371, "Image Out"=w341) -> (w378:T8)
            n138 = Bundle By Name(cluster=cluster{"Command":string, "Data":variant} {"Command"="Average", "Data"=variant} ("element"), "Data"=w378) -> (w380:cluster{"Command":string, "Data":variant})
            n139 = Get Date/Time In Seconds() -> (seconds since 1Jan1904=w366:timestamp)
            n140 = Enqueue Element(queue=w382, element=w380, error in (no error)=w352) -> (error out=w355:errorcluster)  [unwired: 1 in, 2 out]
            n141 = Format Into String(format string="%d of %d ..", initial string="Acquired Dark Image  ", error in=w355, w371, w358) -> (resulting string=w373:string)  [unwired: 1 out]
            n142 = Format Date/Time String(time format string (%c)="%Y-%m-%d  %H:%M:%S    ", seconds (now)=w366) -> (date/time string=w362:string)  [unwired: 1 in]
            n143 = property class="Slide (strict)"(reference=w368, error in=w355, "Caption.Visible"=TRUE, "Caption.Text"=w373) -> (error out=w369:errorcluster)  [unwired: 1 out]
            n144 = Concatenate Strings(w361, w362, "Acquiring Dark Image" ("string"), "\r\n") -> (w360:string)
            n145 = Bundle By Name(cluster=w377, "UI Data.Progress"=w357, "UI Data.Status"=w360, "UI Data.Iteration"=w359) -> (w376:T5)
          }
          frame True {
            w389 = T3[] [enum."Stop Acquisition", enum."Poll", enum."Save Dark Image"] items=["Poll", "Initialize", "Start Acquisition", "Get Dark Image", "Get Bright Image", "Average", "Stop Acquisition", "Save Dark Image", "Save Bright Image", "Error", "Exit"]
            n146 = Get Date/Time In Seconds() -> (seconds since 1Jan1904=w397:timestamp)
            n147 = Format Date/Time String(time format string (%c)="%Y-%m-%d  %H:%M:%S    ", seconds (now)=w397) -> (date/time string=w393:string)  [unwired: 1 in]
            n148 = Concatenate Strings(w394, w393, "Dark Image Averaging Complete.." ("string"), "\r\n") -> (w395:string)
            n149 = Bundle By Name(cluster=w399, "UI Data.Progress"=u16 50, "UI Data.Iteration"=w390, "UI Data.Status"=w395) -> (w398:T5)
          }
        }
      }
      frame "Get Bright Image" {
        n150 = Unbundle By Name(w412) -> ("UI Data.Progress"=w410:u16, "UI Data.Status"=w408:string, "UI Data.Progress 2"=w405:refnum<vi>, "AvgQ"=w407:refnum<queue>, "UI Data.Iteration"=w409:u16, "UI Data.Img Avg Num"=w406:u16, "Image Data.Img  u16 Buffer2"=w403:T4, "Sensor Data.nSensorIP"=w416:string, "Sensor Data.refImg"=w415:u16[], "Sensor Data.pImg"=w414:u16[], "Sensor Data.nHeight"=w413:i32, "Sensor Data.nWidth"=w402:i32, "Sensor Data.Reference Directory"=w401:string)
        n151 = Greater Or Equal?(x=w409, y=w406) -> (x >= y?=w417:bool)
        n152 = case shown="False" w417 {
          tunnel: w419 -> [w466 w479]
          tunnel: [w448 w479] -> w418
          tunnel: w416 -> [w463 _]
          tunnel: w415 -> [w464 _]
          tunnel: w414 -> [w465 _]
          tunnel: w413 -> [w423 _]
          tunnel: w409 -> [w451 w469]
          tunnel: w412 -> [w457 w478]
          tunnel: [w456 w477] -> w411
          tunnel: w410 -> [w437 _]
          tunnel: w408 -> [w440 w473]
          tunnel: w407 -> [w461 _]
          tunnel: w406 -> [w450 _]
          tunnel: w405 -> [w447 _]
          tunnel: [w446 w468] -> w404
          tunnel: w403 -> [w432 _]
          tunnel: w402 -> [w424 _]
          tunnel: w401 -> [w427 _]
          frame False {
            (unwired) cluster{"Iteration":u16, "Image Out":T4} {"Iteration"=0, "Image Out"=refnum}
            w436 = T13 1 items=["ACQ_INIT"=0, "DARK_MODE"=1, "BRIGHT_MODE"=2, "SOFTTRIGGER_MODE"=258, "SOFTTRIGGER_INSTANT_MODE"=259] ("nMode")
            w446 = T3[] [enum."Poll", enum."Get Bright Image"] items=["Poll", "Initialize", "Start Acquisition", "Get Dark Image", "Get Bright Image", "Average", "Stop Acquisition", "Save Dark Image", "Save Bright Image", "Error", "Exit"]
            n153 = call "lvString to lpString.vi"("LVString"=w427) -> ("LPTSTR String"=w425:string)  [unwired: 10 in]
            n154 = Compound Arithmetic op=MULTIPLY(w423, w424, 2 ("value")) -> (w430:i32)
            n155 = To Unsigned Long Integer(number=w430) -> (unsigned 32bit integer=w428:u32)
            n156 = call "BigEndianToLittleEndian_IP.vi"("IP String"=w463) -> ("IP Network Order"=w462:u32)  [unwired: 10 in]
            n157 = String To Byte Array(string=w425) -> (unsigned byte array=w426:u8[])
            n158 = call "Start Continuous Acquisition.vi"("nSensorIP"=w462, "nMode"=w436, "refImg"=w464, "pImg"=w465, "nBuffLength"=w428, "error in (no error)"=w466, "lpszRefPath"=w426) -> ("pImg out"=w422:u16[], "error out"=w434:errorcluster)  [unwired: 5 in, 2 out]
            n159 = Reshape Array(w422, w424, w423) -> (w431:u16[][])
            n160 = call "IMAQ ArrayToImage"("Image Pixels (U16)"=w431, "error in (no error)"=w434, "Image"=w432) -> ("error out"=w433:errorcluster, "Image Out"=w420:T4)  [unwired: 7 in]
            n161 = Bundle By Name(cluster=T8 {"Iteration"=0, "Image Out"=refnum, "pImg"=[]}, "Iteration"=w451, "Image Out"=w420) -> (w458:T8)
            n162 = Increment(x=w451) -> (x+1=w449:u16)
            n163 = Bundle By Name(cluster=cluster{"Command":string, "Data":variant} {"Command"="Average", "Data"=variant} ("element"), "Data"=w458) -> (w459:cluster{"Command":string, "Data":variant})
            n164 = Decrement(x=w450) -> (x-1=w438:u16)
            n165 = Enqueue Element(queue=w461, element=w459, error in (no error)=w433) -> (error out=w435:errorcluster)  [unwired: 1 in, 2 out]
            n166 = Get Date/Time In Seconds() -> (seconds since 1Jan1904=w445:timestamp)
            n167 = Format Into String(format string="%d of %d ..", initial string="Acquired Bright Image  ", error in=w435, w451, w438) -> (resulting string=w453:string)  [unwired: 1 out]
            n168 = Format Date/Time String(time format string (%c)="%Y-%m-%d  %H:%M:%S    ", seconds (now)=w445) -> (date/time string=w441:string)  [unwired: 1 in]
            n169 = property class="Slide (strict)"(reference=w447, error in=w435, "Caption.Visible"=TRUE, "Caption.Text"=w453) -> (error out=w448:errorcluster)  [unwired: 1 out]
            n170 = Concatenate Strings(w440, w441, "Acquiring Bright Image" ("string"), "\r\n") -> (w439:string)
            n171 = Bundle By Name(cluster=w457, "UI Data.Progress"=w437, "UI Data.Status"=w439, "UI Data.Iteration"=w449) -> (w456:T5)
          }
          frame True {
            w468 = T3[] [enum."Stop Acquisition", enum."Poll", enum."Save Bright Image"] items=["Poll", "Initialize", "Start Acquisition", "Get Dark Image", "Get Bright Image", "Average", "Stop Acquisition", "Save Dark Image", "Save Bright Image", "Error", "Exit"]
            n172 = Get Date/Time In Seconds() -> (seconds since 1Jan1904=w476:timestamp)
            n173 = Format Date/Time String(time format string (%c)="%Y-%m-%d  %H:%M:%S    ", seconds (now)=w476) -> (date/time string=w472:string)  [unwired: 1 in]
            n174 = Concatenate Strings(w473, w472, "Bright Image Averaging Complete.." ("string"), "\r\n") -> (w474:string)
            n175 = Bundle By Name(cluster=w478, "UI Data.Progress"=u16 80, "UI Data.Iteration"=w469, "UI Data.Status"=w474) -> (w477:T5)
          }
        }
      }
      frame "Average" {
      }
      frame "Stop Acquisition" {
        n176 = Unbundle By Name(w485) -> ("Sensor Data.nSensorIP"=w484:string)
        n177 = call "BigEndianToLittleEndian_IP.vi"("IP String"=w484) -> ("IP Network Order"=w483:u32)  [unwired: 10 in]
        n178 = call "Stop Continuous Acquisition.vi"("error in (no error)"=w487, "nSensorIP"=w483) -> ("error out"=w486:errorcluster)  [unwired: 8 in, 1 out]
      }
      frame "Save Dark Image" {
        n179 = Unbundle By Name(w507) -> ("AvgQ"=w506:refnum<queue>, "Image Storage Path"=w496:path, "UI Data.Select Image Type"=w501:T1)
        n180 = Get Date/Time In Seconds() -> (seconds since 1Jan1904=w498:timestamp)
        n181 = Format Date/Time String(time format string (%c)="%Y-%m-%d", seconds (now)=w498) -> (date/time string=w495:string)  [unwired: 1 in]
        n182 = Get Date/Time In Seconds() -> (seconds since 1Jan1904=w491:timestamp)
        n183 = Build Path(base path=w496, name or relative path=w495) -> (appended path=w497:path)
        n184 = Format Date/Time String(time format string (%c)="%H_%M_", seconds (now)=w491) -> (date/time string=w489:string)  [unwired: 1 in]
        n185 = call <vilib>:"Check if File or Folder Exists.vi"("error in (no error)"=w500, "path"=w497) -> ("error out"=w488:errorcluster, "file or folder exists?"=w494:bool, "dup path"=w493:path)  [unwired: 7 in]
        n186 = case shown="\"TIFF\", Default" w501 {
          tunnel: [w514 w517] -> w502
          tunnel: w489 -> [w513 w516]
          frame "RAW" {
            n187 = Concatenate Strings(w513, "DarkImage.raw" ("Status")) -> (w514:string)
          }
          frame "TIFF", Default {
            n188 = Concatenate Strings(w516, "DarkImage.tiff" ("Status")) -> (w517:string)
          }
        }
        n189 = case shown="False" w494 {
          tunnel: w493 -> [w510 w512]
          tunnel: [w511 w512] -> w492
          tunnel: w488 -> [w509 _]
          frame False {
            n190 = Create Folder(path (use dialog)=w510, error in=w509) -> (created path=w511:path)  [unwired: 1 in, 2 out]
          }
          frame True {
          }
        }
        n191 = Build Path(base path=w492, name or relative path=w502) -> (appended path=w503:path)
        n192 = Bundle By Name(cluster=cluster{"Command":string, "Data":variant} {"Command"="Save Image", "Data"=variant} ("element"), "Data"=w503) -> (w504:cluster{"Command":string, "Data":variant})
        n193 = Enqueue Element(queue=w506, element=w504, error in (no error)=w500) -> (error out=w508:errorcluster)  [unwired: 1 in, 2 out]
      }
      frame "Save Bright Image" {
        n194 = Unbundle By Name(w538) -> ("AvgQ"=w537:refnum<queue>, "Image Storage Path"=w527:path, "UI Data.Select Image Type"=w532:T1)
        n195 = Get Date/Time In Seconds() -> (seconds since 1Jan1904=w529:timestamp)
        n196 = Format Date/Time String(time format string (%c)="%Y-%m-%d", seconds (now)=w529) -> (date/time string=w526:string)  [unwired: 1 in]
        n197 = Get Date/Time In Seconds() -> (seconds since 1Jan1904=w522:timestamp)
        n198 = Format Date/Time String(time format string (%c)="%H_%M_", seconds (now)=w522) -> (date/time string=w519:string)  [unwired: 1 in]
        n199 = Build Path(base path=w527, name or relative path=w526) -> (appended path=w528:path)
        n200 = call <vilib>:"Check if File or Folder Exists.vi"("error in (no error)"=w531, "path"=w528) -> ("error out"=w520:errorcluster, "file or folder exists?"=w525:bool, "dup path"=w524:path)  [unwired: 7 in]
        n201 = case shown="\"TIFF\", Default" w532 {
          tunnel: [w545 w548] -> w533
          tunnel: w519 -> [w544 w547]
          frame "RAW" {
            n202 = Concatenate Strings(w544, "BrightImage.raw" ("Status")) -> (w545:string)
          }
          frame "TIFF", Default {
            n203 = Concatenate Strings(w547, "BrightImage.tiff" ("Status")) -> (w548:string)
          }
        }
        n204 = case shown="False" w525 {
          tunnel: w524 -> [w541 w543]
          tunnel: [w542 w543] -> w523
          tunnel: w520 -> [w540 _]
          frame False {
            n205 = Create Folder(path (use dialog)=w541, error in=w540) -> (created path=w542:path)  [unwired: 1 in, 2 out]
          }
          frame True {
          }
        }
        n206 = Build Path(base path=w523, name or relative path=w533) -> (appended path=w534:path)
        n207 = Bundle By Name(cluster=cluster{"Command":string, "Data":variant} {"Command"="Save Image", "Data"=variant} ("element"), "Data"=w534) -> (w535:cluster{"Command":string, "Data":variant})
        n208 = Enqueue Element(queue=w537, element=w535, error in (no error)=w531) -> (error out=w539:errorcluster)  [unwired: 1 in, 2 out]
      }
      frame "Error" {
        w551 = u16 0 ("UI Data.Img Avg Num")
        n209 = call <userlib>:"MGI Report Error.vi"("error in"=w554) -> ("no error"=w553:errorcluster)  [unwired: 10 in]
        n210 = Bundle By Name(cluster=w555, "UI Data.Img Avg Num"=w551, "UI Data.Progress"=w551, "UI Data.Status"="") -> (w552:T5)
      }
      frame "Exit" {
        w561 = u16 0 ("UI Data.Progress")
        n211 = Unbundle By Name(w581) -> ("Image Averaging in"=w574:refnum<class "Image Averaging.lvclass">, "Image Averaging in"=w571:refnum<class "Image Averaging.lvclass">, "AvgQ"=w579:refnum<queue>, "UI Data.Progress 2"=w565:refnum<vi>, "Image Data.Img U16 Buffer1"=w557:T4, "Image Data.Img  u16 Buffer2"=w556:T4)
        n212 = Unregister For Events(event registration refnum=w562, error in=w582) -> (error out=w563:errorcluster)
        n213 = call "IMAQ Dispose"("Image"=w556, "error in (no error)"=w563) -> ("error out"=w559:errorcluster)  [unwired: 4 in]
        n214 = call "IMAQ Dispose"("Image"=w557, "error in (no error)"=w559) -> ("error out"=w558:errorcluster)  [unwired: 4 in]
        n215 = property class="Slide (strict)"(reference=w565, error in=w558, "Caption.Text"="Image Averaging Complete..") -> (error out=w568:errorcluster)  [unwired: 1 out]
        n216 = Flush Queue(queue=w579, error in (no error)=w568) -> (queue out=w578:refnum<queue>, error out=w580:errorcluster)  [unwired: 1 out]
        n217 = Enqueue Element At Opposite End(queue=w578, element=cluster{"Command":string, "Data":variant} {"Command"="Exit", "Data"=variant}, error in (no error)=w580) -> (error out=w576:errorcluster)  [unwired: 1 in, 2 out]
        n218 = call <vilib>:"Read Caller Enqueuer.vi"("Actor"=w571) -> ("Caller Enqueuer"=w570:refnum<class "Message Enqueuer.lvclass">)  [unwired: 10 in]
        n219 = call "Send Avg Done.vi"("error in (no error)"=w576, "Message Enqueuer"=w570) -> ("error out"=w572:errorcluster)  [unwired: 8 in, 1 out]
        n220 = call <vilib>:"Read Self Enqueuer.vi"("Actor"=w574) -> ("Self Enqueuer"=w573:refnum<class "Message Enqueuer.lvclass">)  [unwired: 10 in]
        n221 = call <vilib>:"Send Normal Stop.vi"("error in (no error)"=w572, "Message Enqueuer"=w573) -> ("error out"=w575:errorcluster)  [unwired: 9 in]
        n222 = Bundle By Name(cluster=w581, "UI Data.Progress"=w561, "UI Data.Iteration"=w561, "UI Data.Status"="") -> (w569:T5)
        n223 = property class="Slide (strict)"(reference=w565, error in=w575, "Caption.Text"="Progress") -> (error out=w566:errorcluster)  [unwired: 1 out]
      }
    }
    n224 = Unbundle By Name(w189) -> ("UI Data.Progress"=→"Progress":u16, "UI Data.Status Ref"=w186:refnum<vi>, "UI Data.Status"=w185:string)
    n225 = property class="Str"(reference=w186, error in=w192, "Value"=w185, "Text.Scroll Position"=-1) -> (error out=w187:errorcluster)  [unwired: 1 out]
  }
